vi "EvalParsed.vi"(10 "Cluster":T1, 11 "NameSpace":variant) -> (3 "element":dbl)   [LabVIEW 2019, in "Eval.lvlib"]
uses:
  Eval.lvlib
  <vilib>/Utility/Data Type/NI_Data Type.lvlib
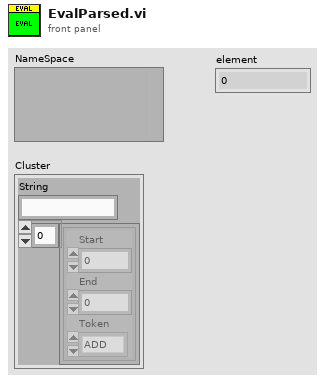
[diagram p1: front panel]
types:
  T1 = cluster{"String":string, cluster{"Start":i32, "End":i32, "Token":enum16{"ADD", "BITAND", "BITOR", "COMMA", "DIV", "Dnumeric", "EQUAL", "EXP", "FUNC", "GREATER", "GREATEREQ", "INumeric", "Identifier", "Ignore", "LESS", "LESSEQ", "LOGAND", "LOGOR", "LPAR", "LSHIFT", "MULT", "N/A", "RPAR", "RSHIFT", "SUB", "UADD", "USUB"}}[]}
  T2 = cluster{"Start":i32, "End":i32, "Token":enum16{"ADD", "BITAND", "BITOR", "COMMA", "DIV", "Dnumeric", "EQUAL", "EXP", "FUNC", "GREATER", "GREATEREQ", "INumeric", "Identifier", "Ignore", "LESS", "LESSEQ", "LOGAND", "LOGOR", "LPAR", "LSHIFT", "MULT", "N/A", "RPAR", "RSHIFT", "SUB", "UADD", "USUB"}}[]
  T3 = enum16{"ADD", "BITAND", "BITOR", "COMMA", "DIV", "Dnumeric", "EQUAL", "EXP", "FUNC", "GREATER", "GREATEREQ", "INumeric", "Identifier", "Ignore", "LESS", "LESSEQ", "LOGAND", "LOGOR", "LPAR", "LSHIFT", "MULT", "N/A", "RPAR", "RSHIFT", "SUB", "UADD", "USUB"}
  T4 = typedef "NI_Data Type.lvlib/Data Type.ctl" = enum8{"Invalid Type", "Void", "I8", "I16", "I32", "I64", "U8", "U16", "U32", "U64", "Single Float", "Double Float", "Extended Float", "Single Complex", "Double Complex", "Extended Complex", "Enum U8", "Enum U16", "Enum U32", "Enum U64", "Single Float With Unit", "Double Float With Unit", "Extended Float With Unit", "Single Complex with Unit", "Double Complex with Unit", "Extended Complex with Unit", "Boolean", "String", "Path", "Picture", "Tag", "Array", "Cluster", "Variant", "LV Variant", "Waveform", "Timestamp", "Digital Waveform", "Digital Data", "ExpressData", "Refnum", "External Data", "VI", "Poly VI", "LabVIEW Class Instance", "Fixed Point", "Set Collection", "Map Collection"}
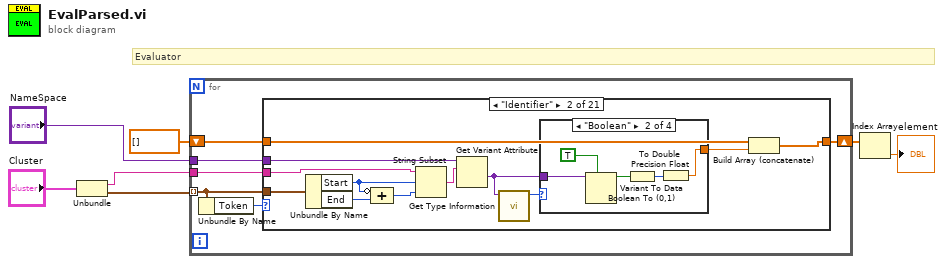
[diagram p0: block diagram]
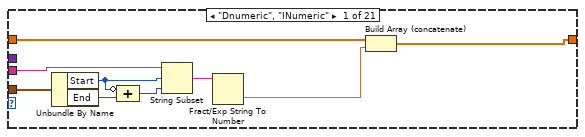
[diagram p2: hidden frame]
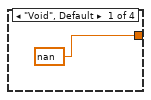
[diagram p3: hidden frame]
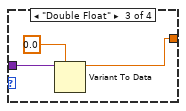
[diagram p4: hidden frame]
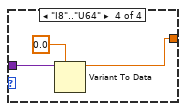
[diagram p5: hidden frame]
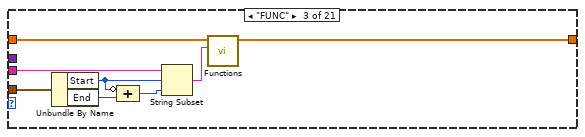
[diagram p6: hidden frame]
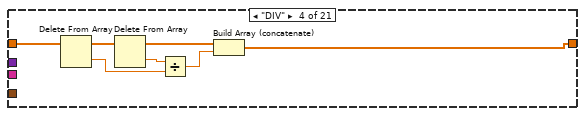
[diagram p7: hidden frame]
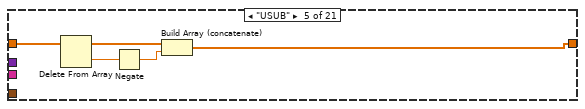
[diagram p8: hidden frame]
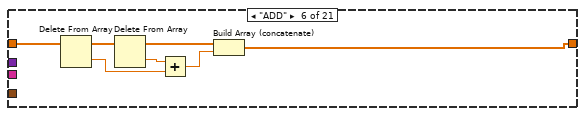
[diagram p9: hidden frame]
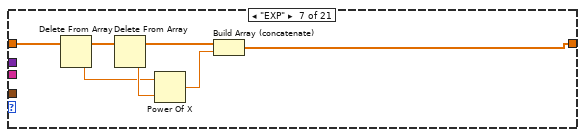
[diagram p10: hidden frame]
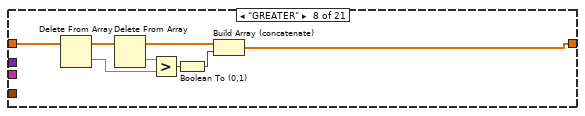
[diagram p11: hidden frame]
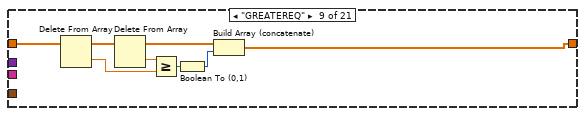
[diagram p12: hidden frame]
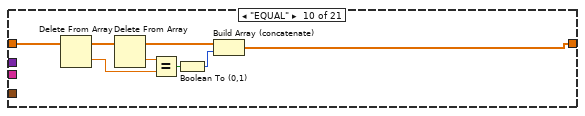
[diagram p13: hidden frame]
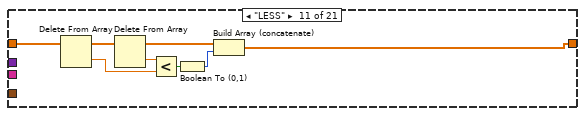
[diagram p14: hidden frame]
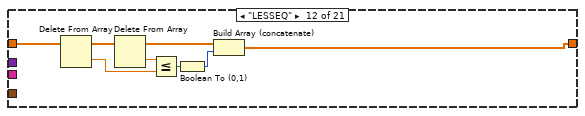
[diagram p15: hidden frame]
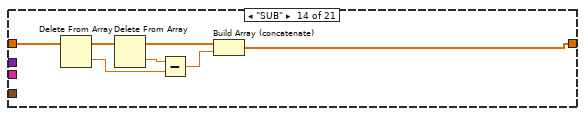
[diagram p17: hidden frame]
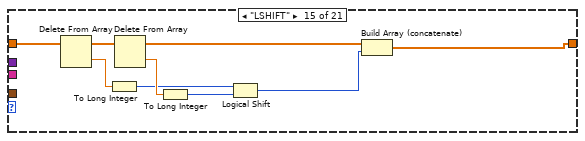
[diagram p18: hidden frame]
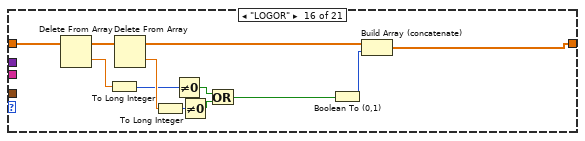
[diagram p19: hidden frame]
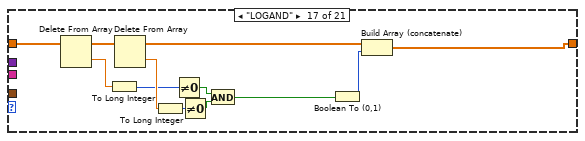
[diagram p20: hidden frame]
diagram:
  # "Evaluator"
  n1 = Unbundle("Cluster") -> ("String"=w5:string, w6:T2)
  n2 = for {
    tunnel: w6 -> [w9] mode=indexing
    shift-right: [w12] -> w4
    shift-left: dbl[] [] -> [w13]
    tunnel: w5 -> [w10]
    tunnel: "NameSpace" -> [w8]
    n3 = Unbundle By Name(w9) -> ("Token"=w11:T3)
    n4 = case shown="\"Identifier\"" w11 {
      tunnel: w13 -> [w22 w34 w49 w61 w66 w73 w80 w88 w96 w104 w112 w120 w121 w128 w137 w149 w161 w170 w179 w189 w196]
      tunnel: [w16 w29 w48 w58 w65 w70 w77 w85 w93 w101 w109 w117 w121 w125 w134 w146 w158 w167 w176 w186 w193] -> w12
      tunnel: w10 -> [w17 w30 w51 _ _ _ _ _ _ _ _ _ _ _ _ _ _ _ _ _ _]
      tunnel: w9 -> [w14 w28 w50 _ _ _ _ _ _ _ _ _ _ _ _ _ _ _ _ _ _]
      tunnel: w8 -> [_ w27 _ _ _ _ _ _ _ _ _ _ _ _ _ _ _ _ _ _ _]
      frame "Dnumeric", "INumeric" {
        n5 = Unbundle By Name(w14) -> ("Start"=w19:i32, "End"=w20:i32)
        n6 = Compound Arithmetic op=ADD(invert w19, w20) -> (w21:i32)
        n7 = String Subset(string=w17, offset (0)=w19, length (rest)=w21) -> (substring=w18:string)
        n8 = Fract/Exp String To Number(string=w18) -> (number=w15:dbl)  [unwired: 3 in, 1 out]
        n9 = Build Array (concatenate)(w22, w15) -> (w16:dbl[])
      }
      frame "Identifier" {
        n10 = Unbundle By Name(w28) -> ("Start"=w31:i32, "End"=w32:i32)
        n11 = Compound Arithmetic op=ADD(invert w31, w32) -> (w33:i32)
        n12 = String Subset(string=w30, offset (0)=w31, length (rest)=w33) -> (substring=w26:string)
        n13 = Get Variant Attribute(Variant=w27, name=w26) -> (value=w24:variant)  [unwired: 2 in, 3 out]
        n14 = call <vilib>:"Get Type Information.vi"("variant"=w24) -> ("type"=w25:T4)  [unwired: 6 in, 4 out]
        n15 = case shown="\"Boolean\"" w25 {
          tunnel: w24 -> [_ w40 w43 w46]
          tunnel: [nan w36 w41 w44] -> w23
          frame "Void", Default {
          }
          frame "Boolean" {
            n16 = Variant To Data(type=TRUE, Variant=w40) -> (data=w38:bool)  [unwired: 1 in, 1 out]
            n17 = Boolean To (0,1)(Boolean=w38) -> (0, 1=w37:i16)
            n18 = To Double Precision Float(number=w37) -> (double precision float=w36:dbl)
          }
          frame "Double Float" {
            n19 = Variant To Data(type=0.0, Variant=w43) -> (data=w41:dbl)  [unwired: 1 in, 1 out]
          }
          frame "I8".."U64" {
            n20 = Variant To Data(type=0.0, Variant=w46) -> (data=w44:dbl)  [unwired: 1 in, 1 out]
          }
        }
        n21 = Build Array (concatenate)(w34, w23) -> (w29:dbl[])
      }
      frame "FUNC" {
        n22 = Unbundle By Name(w50) -> ("Start"=w52:i32, "End"=w53:i32)
        n23 = Compound Arithmetic op=ADD(invert w52, w53) -> (w54:i32)
        n24 = String Subset(string=w51, offset (0)=w52, length (rest)=w54) -> (substring=w47:string)
        n25 = call "Functions.vi"("FUNCTION"=w47, "StackIn"=w49) -> ("StackOut"=w48:dbl[])  [unwired: 9 in]
      }
      frame "DIV" {
        n26 = Delete From Array(array=w61) -> (deleted portion=w56:dbl, array with subset deleted=w60:dbl[])  [unwired: 2 in]
        n27 = Delete From Array(array=w60) -> (deleted portion=w57:dbl, array with subset deleted=w59:dbl[])  [unwired: 2 in]
        n28 = Divide(x=w57, y=w56) -> (x/y=w55:dbl)
        n29 = Build Array (concatenate)(w59, w55) -> (w58:dbl[])
      }
      frame "USUB" {
        n30 = Delete From Array(array=w66) -> (deleted portion=w63:dbl, array with subset deleted=w64:dbl[])  [unwired: 2 in]
        n31 = Negate(x=w63) -> (-x=w62:dbl)
        n32 = Build Array (concatenate)(w64, w62) -> (w65:dbl[])
      }
      frame "ADD" {
        n33 = Delete From Array(array=w73) -> (deleted portion=w68:dbl, array with subset deleted=w72:dbl[])  [unwired: 2 in]
        n34 = Delete From Array(array=w72) -> (deleted portion=w69:dbl, array with subset deleted=w71:dbl[])  [unwired: 2 in]
        n35 = Add(x=w69, y=w68) -> (x+y=w67:dbl)
        n36 = Build Array (concatenate)(w71, w67) -> (w70:dbl[])
      }
      frame "EXP" {
        n37 = Delete From Array(array=w80) -> (deleted portion=w74:dbl, array with subset deleted=w79:dbl[])  [unwired: 2 in]
        n38 = Delete From Array(array=w79) -> (deleted portion=w75:dbl, array with subset deleted=w78:dbl[])  [unwired: 2 in]
        n39 = Power Of X(1:w75, 2:w74) -> (0:w76:dbl)
        n40 = Build Array (concatenate)(w78, w76) -> (w77:dbl[])
      }
      frame "GREATER" {
        n41 = Delete From Array(array=w88) -> (deleted portion=w83:dbl, array with subset deleted=w87:dbl[])  [unwired: 2 in]
        n42 = Delete From Array(array=w87) -> (deleted portion=w84:dbl, array with subset deleted=w86:dbl[])  [unwired: 2 in]
        n43 = Greater?(x=w84, y=w83) -> (0:w82:bool)
        n44 = Boolean To (0,1)(Boolean=w82) -> (0, 1=w81:i16)
        n45 = Build Array (concatenate)(w86, w81) -> (w85:dbl[])
      }
      frame "GREATEREQ" {
        n46 = Delete From Array(array=w96) -> (deleted portion=w91:dbl, array with subset deleted=w95:dbl[])  [unwired: 2 in]
        n47 = Delete From Array(array=w95) -> (deleted portion=w92:dbl, array with subset deleted=w94:dbl[])  [unwired: 2 in]
        n48 = Greater Or Equal?(x=w92, y=w91) -> (x >= y?=w90:bool)
        n49 = Boolean To (0,1)(Boolean=w90) -> (0, 1=w89:i16)
        n50 = Build Array (concatenate)(w94, w89) -> (w93:dbl[])
      }
      frame "EQUAL" {
        n51 = Delete From Array(array=w104) -> (deleted portion=w99:dbl, array with subset deleted=w103:dbl[])  [unwired: 2 in]
        n52 = Delete From Array(array=w103) -> (deleted portion=w100:dbl, array with subset deleted=w102:dbl[])  [unwired: 2 in]
        n53 = Equal?(x=w100, y=w99) -> (x = y?=w98:bool)
        n54 = Boolean To (0,1)(Boolean=w98) -> (0, 1=w97:i16)
        n55 = Build Array (concatenate)(w102, w97) -> (w101:dbl[])
      }
      frame "LESS" {
        n56 = Delete From Array(array=w112) -> (deleted portion=w107:dbl, array with subset deleted=w111:dbl[])  [unwired: 2 in]
        n57 = Delete From Array(array=w111) -> (deleted portion=w108:dbl, array with subset deleted=w110:dbl[])  [unwired: 2 in]
        n58 = Less?(x=w108, y=w107) -> (x < y?=w106:bool)
        n59 = Boolean To (0,1)(Boolean=w106) -> (0, 1=w105:i16)
        n60 = Build Array (concatenate)(w110, w105) -> (w109:dbl[])
      }
      frame "LESSEQ" {
        n61 = Delete From Array(array=w120) -> (deleted portion=w115:dbl, array with subset deleted=w119:dbl[])  [unwired: 2 in]
        n62 = Delete From Array(array=w119) -> (deleted portion=w116:dbl, array with subset deleted=w118:dbl[])  [unwired: 2 in]
        n63 = Less Or Equal?(x=w116, y=w115) -> (x <= y?=w114:bool)
        n64 = Boolean To (0,1)(Boolean=w114) -> (0, 1=w113:i16)
        n65 = Build Array (concatenate)(w118, w113) -> (w117:dbl[])
      }
      frame Default {
      }
      frame "SUB" {
        n66 = Delete From Array(array=w128) -> (deleted portion=w123:dbl, array with subset deleted=w127:dbl[])  [unwired: 2 in]
        n67 = Delete From Array(array=w127) -> (deleted portion=w124:dbl, array with subset deleted=w126:dbl[])  [unwired: 2 in]
        n68 = Subtract(x=w124, y=w123) -> (x-y=w122:dbl)
        n69 = Build Array (concatenate)(w126, w122) -> (w125:dbl[])
      }
      frame "LSHIFT" {
        n70 = Delete From Array(array=w137) -> (deleted portion=w132:dbl, array with subset deleted=w136:dbl[])  [unwired: 2 in]
        n71 = To Long Integer(number=w132) -> (32bit integer=w129:i32)
        n72 = Delete From Array(array=w136) -> (deleted portion=w133:dbl, array with subset deleted=w135:dbl[])  [unwired: 2 in]
        n73 = To Long Integer(number=w133) -> (32bit integer=w130:i32)
        n74 = Logical Shift(y=w129, x=w130) -> (x << y=w131:i32)
        n75 = Build Array (concatenate)(w135, w131) -> (w134:dbl[])
      }
      frame "LOGOR" {
        n76 = Delete From Array(array=w149) -> (deleted portion=w144:dbl, array with subset deleted=w148:dbl[])  [unwired: 2 in]
        n77 = To Long Integer(number=w144) -> (32bit integer=w143:i32)
        n78 = Delete From Array(array=w148) -> (deleted portion=w145:dbl, array with subset deleted=w147:dbl[])  [unwired: 2 in]
        n79 = To Long Integer(number=w145) -> (32bit integer=w142:i32)
        n80 = Not Equal To 0?(x=w143) -> (x != 0?=w140:bool)
        n81 = Not Equal To 0?(x=w142) -> (x != 0?=w141:bool)
        n82 = Or(x=w140, y=w141) -> (x .or. y?=w139:bool)
        n83 = Boolean To (0,1)(Boolean=w139) -> (0, 1=w138:i16)
        n84 = Build Array (concatenate)(w147, w138) -> (w146:dbl[])
      }
      frame "LOGAND" {
        n85 = Delete From Array(array=w161) -> (deleted portion=w156:dbl, array with subset deleted=w160:dbl[])  [unwired: 2 in]
        n86 = To Long Integer(number=w156) -> (32bit integer=w155:i32)
        n87 = Delete From Array(array=w160) -> (deleted portion=w157:dbl, array with subset deleted=w159:dbl[])  [unwired: 2 in]
        n88 = To Long Integer(number=w157) -> (32bit integer=w154:i32)
        n89 = Not Equal To 0?(x=w155) -> (x != 0?=w152:bool)
        n90 = Not Equal To 0?(x=w154) -> (x != 0?=w153:bool)
        n91 = And(x=w152, y=w153) -> (x .and. y?=w151:bool)
        n92 = Boolean To (0,1)(Boolean=w151) -> (0, 1=w150:i16)
        n93 = Build Array (concatenate)(w159, w150) -> (w158:dbl[])
      }
      frame "BITOR" {
        n94 = Delete From Array(array=w170) -> (deleted portion=w165:dbl, array with subset deleted=w169:dbl[])  [unwired: 2 in]
        n95 = To Long Integer(number=w165) -> (32bit integer=w163:i32)
        n96 = Delete From Array(array=w169) -> (deleted portion=w166:dbl, array with subset deleted=w168:dbl[])  [unwired: 2 in]
        n97 = To Long Integer(number=w166) -> (32bit integer=w164:i32)
        n98 = Or(x=w163, y=w164) -> (x .or. y?=w162:i32)
        n99 = Build Array (concatenate)(w168, w162) -> (w167:dbl[])
      }
      frame "BITAND" {
        n100 = Delete From Array(array=w179) -> (deleted portion=w174:dbl, array with subset deleted=w178:dbl[])  [unwired: 2 in]
        n101 = To Long Integer(number=w174) -> (32bit integer=w172:i32)
        n102 = Delete From Array(array=w178) -> (deleted portion=w175:dbl, array with subset deleted=w177:dbl[])  [unwired: 2 in]
        n103 = To Long Integer(number=w175) -> (32bit integer=w173:i32)
        n104 = And(x=w172, y=w173) -> (x .and. y?=w171:i32)
        n105 = Build Array (concatenate)(w177, w171) -> (w176:dbl[])
      }
      frame "RSHIFT" {
        n106 = Delete From Array(array=w189) -> (deleted portion=w184:dbl, array with subset deleted=w188:dbl[])  [unwired: 2 in]
        n107 = To Long Integer(number=w184) -> (32bit integer=w181:i32)
        n108 = Delete From Array(array=w188) -> (deleted portion=w185:dbl, array with subset deleted=w187:dbl[])  [unwired: 2 in]
        n109 = To Long Integer(number=w185) -> (32bit integer=w182:i32)
        n110 = Negate(x=w181) -> (-x=w180:i32)
        n111 = Logical Shift(y=w180, x=w182) -> (x << y=w183:i32)
        n112 = Build Array (concatenate)(w187, w183) -> (w186:dbl[])
      }
      frame "MULT" {
        n113 = Delete From Array(array=w196) -> (deleted portion=w191:dbl, array with subset deleted=w195:dbl[])  [unwired: 2 in]
        n114 = Delete From Array(array=w195) -> (deleted portion=w192:dbl, array with subset deleted=w194:dbl[])  [unwired: 2 in]
        n115 = Multiply(x=w192, y=w191) -> (x*y=w190:dbl)
        n116 = Build Array (concatenate)(w194, w190) -> (w193:dbl[])
      }
    }
  }
  n117 = Index Array(array=w4) -> (element=→"element":dbl)  [unwired: 1 in]
